vi "Load Subitems.vi"(7 "defer fp updates?(T)":bool=TRUE, 8 "error in (no error)":errorcluster, 9 "Tag":string, 11 "Application Data in":T1) -> (0 "error out":errorcluster, 1 "item children":string[](array[string]), 3 "Application Data out":T1)   [LabVIEW 2017, in "DSF Core.lvlib"]
uses:
  DSF Core.lvlib
  Main VI/Application Data.ctl
  <vilib>/NI/Memory Manager/Classes/Pointer/Pointer.lvclass
  Classes/Framework/Framework.lvclass
  Buffer Reader/Buffer Data.ctl
  Classes/Buffer/Buffer.lvclass
  Classes/Transfer Group Status/Status.lvclass
  Typedefs/DSF Engine Framework Configuration.ctl
  Typedefs/DSF Engine Plugin Configuration.ctl
  Typedefs/DSF Timing Info.ctl
  Typedefs/DSF Engine Plugin Thread Configuration.ctl
  Typedefs/DSF Settings Info.ctl
  Typedefs/DSF Engine Transfer Group Configuration.ctl
  Typedefs/DSF Direction.ctl
  Typedefs/DSF Engine Transfer Configuration.ctl
  Typedefs/DSF Byte Order.ctl
  Typedefs/DSF Engine Channel Configuration.ctl
  Typedefs/DSF Data Type.ctl
  Typedefs/DSF Timeout Behavior.ctl
  Classes/Configuration/Configuration Session.lvclass
  Classes/Configuration/Read Plugin.vi
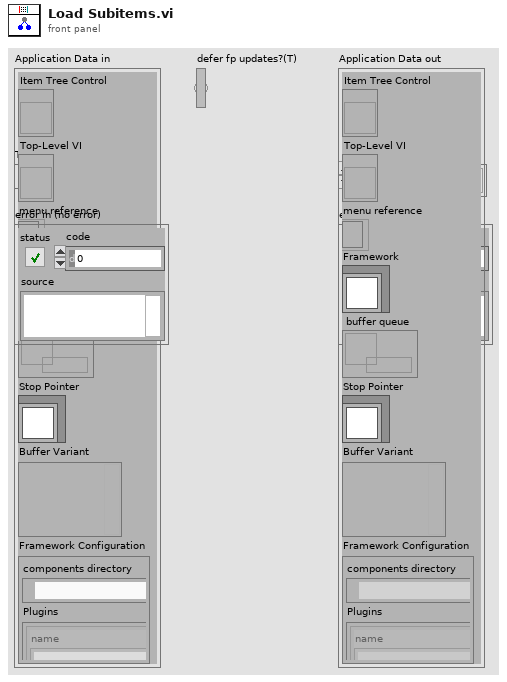
[diagram p1: front panel]
types:
  T1 = typedef "DSF Core.lvlib/Application Data.ctl" = cluster{"Item Tree Control":refnum<vi>, "Top-Level VI":refnum<vi>, "menu reference":refnum<k9>, "Framework":refnum<class "Framework.lvclass">, "buffer queue":refnum<queue>, "Stop Pointer":refnum<class "Pointer.lvclass">, "Buffer Variant":variant, "Framework Configuration":T2}
  T2 = typedef "DSF Core.lvlib/DSF Engine Framework Configuration.ctl" = cluster{"components directory":path, "Plugins":T3[]}
  T3 = typedef "DSF Core.lvlib/DSF Engine Plugin Configuration.ctl" = cluster{"name":string, "components":string[], "cycle timing":T4, "threads":T5[], "Transfer Groups":T7[], "settings":T6}
  T4 = typedef "DSF Core.lvlib/DSF Timing Info.ctl" = cluster{"priority":u64, "decimation":u64, "offset":u64}
  T5 = typedef "DSF Core.lvlib/DSF Engine Plugin Thread Configuration.ctl" = cluster{"buffer converter settings":T6, "transceiver settings":T6, "processor":i32, "priority offset":i16}
  T6 = typedef "DSF Core.lvlib/DSF Settings Info.ctl" = cluster{"key":string, "value":string}[]
  T7 = typedef "DSF Core.lvlib/DSF Engine Transfer Group Configuration.ctl" = cluster{"name":string, "direction":T8, "cycle timing":T4, "thread index":i32, "settings":T6, "Transfers":T9[], "timeout behavior":T13}
  T8 = typedef "DSF Core.lvlib/DSF Direction.ctl" = enum8{"Tx", "Rx"}
  T9 = typedef "DSF Core.lvlib/DSF Engine Transfer Configuration.ctl" = cluster{"name":string, "byte order":T10, "settings":T6, "channels":T11[]}
  T10 = typedef "DSF Core.lvlib/DSF Byte Order.ctl" = enum8{"big-endian", "little-endian"}
  T11 = typedef "DSF Core.lvlib/DSF Engine Channel Configuration.ctl" = cluster{"string offset":u64, "string data type":T12, "engine data type":T12, "name":string, "settings":T6}
  T12 = typedef "DSF Core.lvlib/DSF Data Type.ctl" = enum8{"Bool", "SGL", "DBL", "I8", "I16", "I32", "I64", "U8", "U16", "U32", "U64"}
  T13 = typedef "DSF Core.lvlib/DSF Timeout Behavior.ctl" = enum8{"Increment Late Count", "Throw Error"}
  T14 = typedef "DSF Core.lvlib/Tree Item Type.ctl" = enum16{"Framework", "Plugin Group", "Plugin", "Group", "Transfer", "Buffer", "Channel"}
  T15 = typedef "DSF Core.lvlib/DSF Plugin Info.ctl" = cluster{"components":string[], "timing":T4, "group ids":string[], "settings id":string, "threads":T5[]}
  T16 = typedef "DSF Core.lvlib/Tree Item.ctl" = cluster{"Left Cell String":string, "Child Text":string[], "Child Tag":string, "Glyph Index":i32}
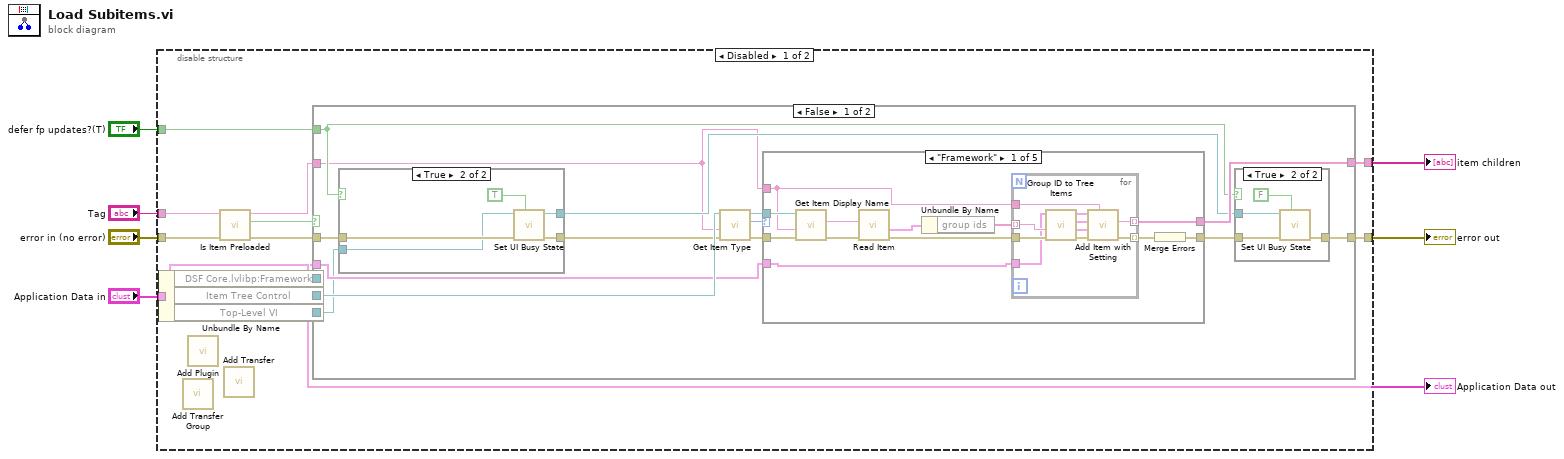
[diagram p0: block diagram]
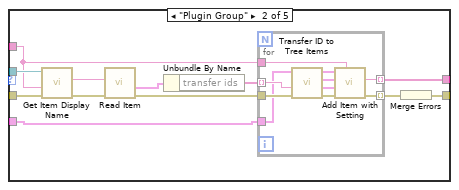
[diagram p4: hidden frame]
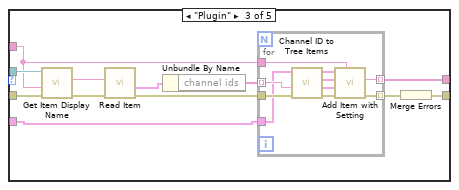
[diagram p5: hidden frame]
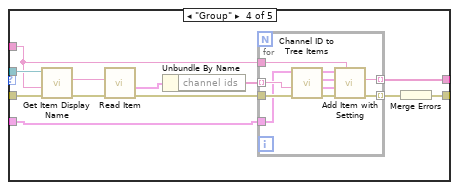
[diagram p6: hidden frame]
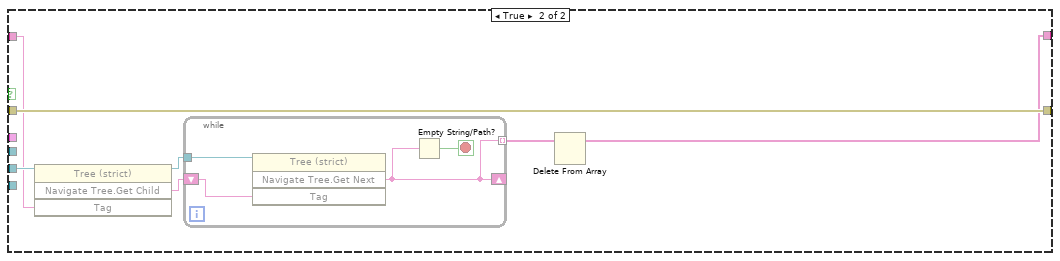
[diagram p8: hidden frame]
diagram:
  n1 = disable-structure shown="Disabled" {
    disable-tunnel: "Tag" -> [w16 _]
    disable-tunnel: [w14 _] -> w5
    disable-tunnel: "error in (no error)" -> [w13 _]
    disable-tunnel: [w12 _] -> w3
    disable-tunnel: "Application Data in" -> [w10 _]
    disable-tunnel: "defer fp updates?(T)" -> [w8 _]
    frame Disabled {
      n2 = Unbundle By Name(w10) -> ("DSF Core.lvlibp:Framework"=w7:refnum<class "Framework.lvclass">, "Item Tree Control"=w11:refnum<vi>, "Top-Level VI"=w9:refnum<vi>)
      n3 = call "Add Transfer Group.vi"() -> ()  [unwired: 9 in, 3 out]
      n4 = call "Add Plugin.vi"() -> ()  [unwired: 9 in, 3 out]
      n5 = call "Is Item Preloaded"("error in (no error)"=w13, "Tag in"=w16) -> ("error out"=w15:errorcluster, "replaced"=w17:bool, "Tag out"=w18:string)  [unwired: 7 in]
      n6 = call "Add Transfer.vi"() -> ()  [unwired: 10 in, 2 out]
      n7 = case shown="False" w17 {
        tunnel: w11 -> [w29 w138]
        tunnel: [w22 w139] -> w14
        tunnel: w15 -> [w28 w139]
        tunnel: w18 -> [w19 w137]
        tunnel: [w27 w134] -> w12
        tunnel: w10 -> [w25 _]
        tunnel: w9 -> [w24 _]
        tunnel: w8 -> [w20 _]
        tunnel: w7 -> [_ _]
        frame False {
          n8 = case shown="True" w20 {
            tunnel: w28 -> [w38 w43]
            tunnel: w24 -> [_ w42]
            tunnel: [w38 w41] -> w23
            tunnel: [_ w40] -> w21
            frame False {
            }
            frame True {
              n9 = call "Set UI Busy State.vi"("Defer Panel Updates"=TRUE, "error in (no error)"=w43, "VI in"=w42) -> ("error out"=w41:errorcluster, "VI out"=w40:refnum<vi>)  [unwired: 7 in]
            }
          }
          n10 = call "Get Item Type.vi"("error in (no error)"=w23, "Tag"=w19, "TreeControl in"=w29) -> ("error out"=w32:errorcluster, "Item Type"=w31:T14, "TreeControl out"=w26:refnum<vi>)  [unwired: 6 in]
          n11 = case shown="\"Framework\"" w31 {
            tunnel: w26 -> [w55 w77 w99 w121 _]
            tunnel: w32 -> [w54 w76 w98 w120 w132]
            tunnel: [w48 w71 w94 w116 w132] -> w30
            tunnel: w19 -> [w45 w67 w89 w111 _]
            tunnel: [w47 w69 w91 w113 _] -> w27
            tunnel: w25 -> [w46 w68 w90 w112 _]
            frame "Framework" {
              n12 = call "Get Item Display Name.vi"("error in (no error)"=w54, "Tag"=w45, "TreeControl in"=w55) -> ("error out"=w53:errorcluster, "display name"=w44:string)  [unwired: 6 in, 1 out]
              n13 = call-poly "Read Item.vi"("error in (no error)"=w53, "Plugin ID"=w44) -> ("error out"=w50:errorcluster, "value"=w52:T15)  [unwired: 6 in, 2 out]
              n14 = Unbundle By Name(w52) -> ("group ids"=w51:string[])
              n15 = for {
                tunnel: w51 -> [w65] mode=indexing
                tunnel: w50 -> [w64]
                tunnel: [w62] -> w49 mode=indexing
                tunnel: w45 -> [w57]
                tunnel: [w60] -> w47 mode=indexing
                tunnel: w46 -> [w59]
                n16 = call "Group ID to Tree Items.vi"("error in (no error)"=w64, "Group ID"=w65, "Application Data in"=w59) -> ("error out"=w63:errorcluster, "Settings"=w56:T16, "Item"=w61:T16, "Application Data out"=w58:T1)  [unwired: 5 in]
                n17 = call "Add Item with Setting.vi"("Tag"=w57, "error in (no error)"=w63, "Setting"=w56, "Item"=w61, "Application Data in"=w58) -> ("error out"=w62:errorcluster, "new item tag"=w60:string)  [unwired: 4 in, 1 out]
              }
              n18 = Merge Errors(w49) -> (w48:errorcluster)
            }
            frame "Plugin Group" {
              n19 = call "Get Item Display Name.vi"("error in (no error)"=w76, "Tag"=w67, "TreeControl in"=w77) -> ("error out"=w75:errorcluster, "display name"=w66:string)  [unwired: 6 in, 1 out]
              n20 = call-poly "Read Item.vi"("error in (no error)"=w75, "Plugin ID"=w66) -> ("error out"=w72:errorcluster, "value"=w74:T15)  [unwired: 6 in, 2 out]
              n21 = Unbundle By Name(w74) -> ("transfer ids"=w73:string[])
              n22 = for {
                tunnel: w73 -> [w87] mode=indexing
                tunnel: w72 -> [w86]
                tunnel: [w84] -> w70 mode=indexing
                tunnel: w67 -> [w80]
                tunnel: [w83] -> w69 mode=indexing
                tunnel: w68 -> [w81]
                n23 = call "Transfer ID to Tree Items.vi"("error in (no error)"=w86, "Transfer ID"=w87, "Application Data in"=w81) -> ("error out"=w85:errorcluster, "Settings"=w78:T16, "Item"=w79:T16, "Application Data out"=w82:T1)  [unwired: 5 in]
                n24 = call "Add Item with Setting.vi"("Tag"=w80, "error in (no error)"=w85, "Setting"=w78, "Item"=w79, "Application Data in"=w82) -> ("error out"=w84:errorcluster, "new item tag"=w83:string)  [unwired: 4 in, 1 out]
              }
              n25 = Merge Errors(w70) -> (w71:errorcluster)
            }
            frame "Plugin" {
              n26 = call "Get Item Display Name.vi"("error in (no error)"=w98, "Tag"=w89, "TreeControl in"=w99) -> ("error out"=w97:errorcluster, "display name"=w88:string)  [unwired: 6 in, 1 out]
              n27 = call-poly "Read Item.vi"("error in (no error)"=w97, "Plugin ID"=w88) -> ("error out"=w95:errorcluster, "value"=w96:T15)  [unwired: 6 in, 2 out]
              n28 = Unbundle By Name(w96) -> ("channel ids"=w92:string[])
              n29 = for {
                tunnel: w92 -> [w109] mode=indexing
                tunnel: w95 -> [w108]
                tunnel: [w106] -> w93 mode=indexing
                tunnel: w89 -> [w102]
                tunnel: [w105] -> w91 mode=indexing
                tunnel: w90 -> [w104]
                n30 = call "Channel ID to Tree Items.vi"("error in (no error)"=w108, "Channel ID"=w109, "Application Data in"=w104) -> ("error out"=w107:errorcluster, "Settings"=w101:T16, "Item"=w100:T16, "Application Data out"=w103:T1)  [unwired: 5 in]
                n31 = call "Add Item with Setting.vi"("Tag"=w102, "error in (no error)"=w107, "Setting"=w101, "Item"=w100, "Application Data in"=w103) -> ("error out"=w106:errorcluster, "new item tag"=w105:string)  [unwired: 4 in, 1 out]
              }
              n32 = Merge Errors(w93) -> (w94:errorcluster)
            }
            frame "Group" {
              n33 = call "Get Item Display Name.vi"("error in (no error)"=w120, "Tag"=w111, "TreeControl in"=w121) -> ("error out"=w119:errorcluster, "display name"=w110:string)  [unwired: 6 in, 1 out]
              n34 = call-poly "Read Item.vi"("error in (no error)"=w119, "Plugin ID"=w110) -> ("error out"=w117:errorcluster, "value"=w118:T15)  [unwired: 6 in, 2 out]
              n35 = Unbundle By Name(w118) -> ("channel ids"=w114:string[])
              n36 = for {
                tunnel: w114 -> [w131] mode=indexing
                tunnel: w117 -> [w130]
                tunnel: [w128] -> w115 mode=indexing
                tunnel: w111 -> [w124]
                tunnel: [w127] -> w113 mode=indexing
                tunnel: w112 -> [w126]
                n37 = call "Channel ID to Tree Items.vi"("error in (no error)"=w130, "Channel ID"=w131, "Application Data in"=w126) -> ("error out"=w129:errorcluster, "Settings"=w123:T16, "Item"=w122:T16, "Application Data out"=w125:T1)  [unwired: 5 in]
                n38 = call "Add Item with Setting.vi"("Tag"=w124, "error in (no error)"=w129, "Setting"=w123, "Item"=w122, "Application Data in"=w125) -> ("error out"=w128:errorcluster, "new item tag"=w127:string)  [unwired: 4 in, 1 out]
              }
              n39 = Merge Errors(w115) -> (w116:errorcluster)
            }
            frame "Transfer" {
            }
          }
          n40 = case shown="True" w20 {
            tunnel: w30 -> [w33 w37]
            tunnel: [w33 w36] -> w22
            tunnel: w21 -> [_ w35]
            frame False {
            }
            frame True {
              n41 = call "Set UI Busy State.vi"("Defer Panel Updates"=FALSE, "error in (no error)"=w37, "VI in"=w35) -> ("error out"=w36:errorcluster)  [unwired: 7 in, 1 out]
            }
          }
        }
        frame True {
          n42 = invoke class="Tree (strict)" method="Navigate Tree.Get Child"(reference=w138, "Tag"=w137) -> (reference out=w136:refnum<vi>, "Navigate Tree:Get Child"=w133:string)  [unwired: 2 in, 2 out]
          n43 = while {
            tunnel: w136 -> [w143]
            tunnel: [w140] -> w135 mode=indexing
            shift-right: [w140] -> _
            shift-left: w133 -> [w141]
            stop <- w142 stop-if-true
            n44 = invoke class="Tree (strict)" method="Navigate Tree.Get Next"(reference=w143, "Tag"=w141) -> ("Navigate Tree:Get Next Item"=w140:string)  [unwired: 2 in, 3 out]
            n45 = Empty String/Path?(string/path=w140) -> (empty?=w142:bool)
          }
          n46 = Delete From Array(array=w135) -> (array with subset deleted=w134:string[])  [unwired: 2 in, 1 out]
        }
      }
    }
    frame Enabled {
    }
  }
  "error out" <- w5
  "item children" <- w3
  "Application Data out" <- "Application Data in"
